vi "Color Sensor V3 Initialize.vi"(8 "error in (no error)":errorcluster, 11 "ColorSensorDevRef":T1={"I2CDevRef"={"DevStatus"={"status"=FALSE, "code"=0, "source"=""}, "Device Address"=0, "Handle"=0, "I2C Bus"=enum."Invalid"}} {"I2CDevRef"."Device Address" format="%.0x"}) -> (0 "error out":errorcluster, 3 "ColorSensorDevRef out":T1={"I2CDevRef"={"DevStatus"={"status"=FALSE, "code"=0, "source"=""}, "Device Address"=0, "Handle"=0, "I2C Bus"=enum."Invalid"}} {"I2CDevRef"."Device Address" format="%.0x"})   [LabVIEW 2023]
uses:
  Typedef/Color Sensor V3 DevRef.ctl
  <vilib>/Rock Robotics/WPI/I2C/WPI_I2CDevRef.ctl
  <vilib>/Rock Robotics/SystemInterfaces/i2clib/i2c_bus.ctl
  Typedef/Color Sensor V3 LEDPulseFreq.ctl
  Typedef/Color Sensor V3 LEDCurrent.ctl
  Typedef/Color Sensor V3 ProxResolution.ctl
  Typedef/Color Sensor V3 ProximityRate.ctl
  Typedef/Color Sensor V3 Resolution.ctl
  Typedef/Color Sensor V3 MeasurementRate.ctl
  Typedef/Color Sensor V3 GainFactor.ctl
  Typedef/Color Sensor V3 Registers.ctl
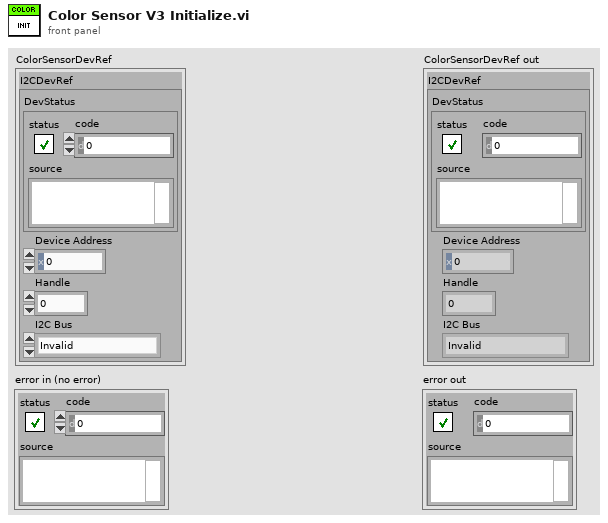
[diagram p1: front panel]
types:
  T1 = typedef "Color Sensor V3 DevRef.ctl" = cluster{"I2CDevRef":T2}
  T2 = typedef "WPI_I2CDevRef.ctl" = cluster{"DevStatus":errorcluster, "Device Address":u8, "Handle":i32, "I2C Bus":T3}
  T3 = typedef "i2c_bus.ctl" = enum16{"I2C On-Board", "I2C MXP", "Invalid"}
  T4 = typedef "Color Sensor V3 Registers.ctl" = enum16{"MainCtrl", "ProximitSensorLED", "ProximitySensorPulse", "ProximitySensorRate", "LightSensorMeasurementRate", "LightSensorGainRegister", "PartIDRegister", "MainStatus", "ProximityData", "ProximityData1", "InfraredData", "InfraredData1", "InfraredData2", "GreenData", "GreenData1", "GreenData2", "BlueData", "BlueData1", "BlueData2", "RedData", "RedData1", "RedData2"}
  T5 = typedef "Color Sensor V3 GainFactor.ctl" = enum16{"1x", "3x", "6x", "9x", "18x"}
  T6 = typedef "Color Sensor V3 MeasurementRate.ctl" = enum16{"25ms", "50ms", "100ms", "200ms", "500ms", "1000ms", "2000ms"}
  T7 = typedef "Color Sensor V3 Resolution.ctl" = enum16{"20bit", "19bit", "18bit", "17bit", "16bit", "13bit"}
  T8 = typedef "Color Sensor V3 ProximityRate.ctl" = enum16{"6ms", "12ms", "25ms", "50ms", "100ms", "200ms", "400ms"}
  T9 = typedef "Color Sensor V3 ProxResolution.ctl" = enum8{"8bit", "9bit", "10bit", "11bit"}
  T10 = typedef "Color Sensor V3 LEDCurrent.ctl" = enum8{"2.5mA", "5.0mA", "10mA", "25mA", "50mA", "75mA", "100mA", "125mA"}
  T11 = typedef "Color Sensor V3 LEDPulseFreq.ctl" = enum16{"60kHz", "70kHz", "80kHz", "90kHz", "100kHz"}
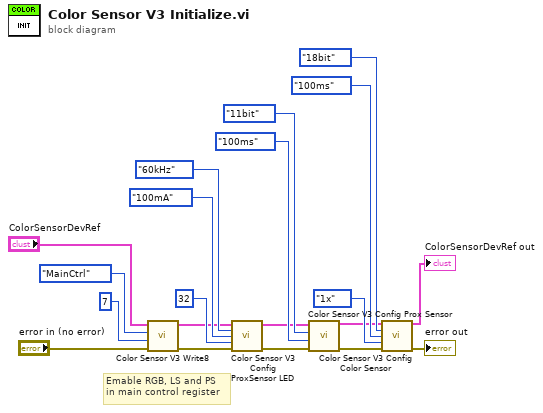
[diagram p0: block diagram]
diagram:
  # "Emable RGB, LS and PS\nin main control register"
  n1 = call "Color Sensor V3 Write8.vi"("error in (no error)"="error in (no error)", "Data"=u8 7, "Registers"=Color_Sensor_V3_Registers."MainCtrl", "ColorSensorDevRef"="ColorSensorDevRef") -> ("error out"=w1:errorcluster, "ColorSensorDevRef out"=w2:T1)  [unwired: 6 in]
  n2 = call "Color Sensor V3 Config ProxSensor LED.vi"("ColorSensorDevRef"=w2, "LEDPulseFreq"=Color_Sensor_V3_LEDPulseFreq."60kHz", "LEDCurrent"=Color_Sensor_V3_LEDCurrent."100mA", "Pulses"=u8 32, "error in (no error)"=w1) -> ("ColorSensorDevRef out"=w14:T1, "error out"=w15:errorcluster)  [unwired: 9 in]
  n3 = call "Color Sensor V3 Config Prox Sensor.vi"("error in (no error)"=w15, "ProximitySensorMeasurementRate"=Color_Sensor_V3_ProximityRate."100ms", "ProximitySensorResolution"=Color_Sensor_V3_ProxResolution."11bit", "ColorSensorDevRef"=w14) -> ("error out"=w9:errorcluster, "ColorSensorDevRef out"=w10:T1)  [unwired: 6 in]
  n4 = call "Color Sensor V3 Config Color Sensor.vi"("ColorSensorDevRef"=w10, "ColorSensorResolution"=Color_Sensor_V3_Resolution."18bit", "ColorSensorMeasurementRate"=Color_Sensor_V3_MeasurementRate."100ms", "GainFactor"=Color_Sensor_V3_GainFactor."1x", "error in (no error)"=w9) -> ("ColorSensorDevRef out"=→"ColorSensorDevRef out":T1, "error out"=→"error out":errorcluster)  [unwired: 9 in]
